vi "WPI_CAN_PDPGlobal.vi"(7 "Write After Receive":T2, 8 "Command":bool, 10 "Operation":T3, 11 "Power Distribution Panel (0)":u8) -> (0 "Commands":T1, 1 "Get All":T2, 3 "Power Distribution Panel Out":u8)   [LabVIEW 2017]
uses:
  <vilib>/Rock Robotics/WPI/CAN/PDP/WPI_CAN_PDPGlobalOps.ctl
  <vilib>/Rock Robotics/WPI/CAN/PDP/WPI_CAN_PDPGetAll.ctl
  <vilib>/Rock Robotics/WPI/CAN/PDP/WPI_CAN_PDPCommands.ctl
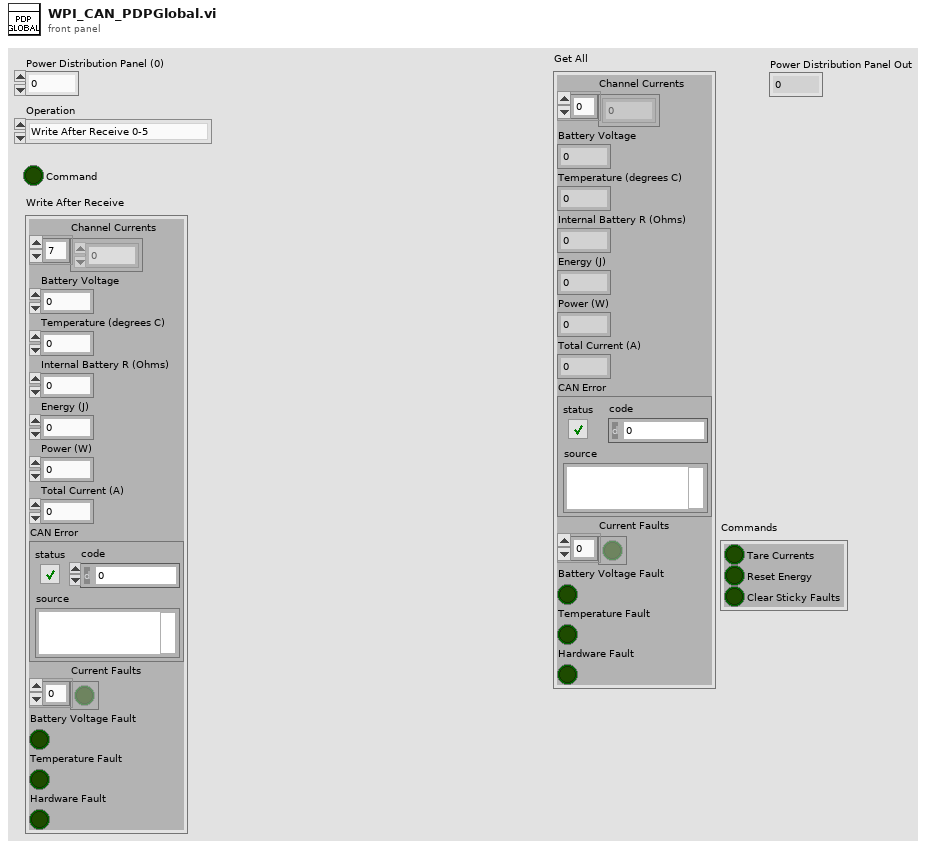
[diagram p1: front panel]
types:
  T1 = typedef "WPI_CAN_PDPCommands.ctl" = cluster{"Tare Currents":bool, "Reset Energy":bool, "Clear Sticky Faults":bool}
  T2 = typedef "WPI_CAN_PDPGetAll.ctl" = cluster{"Channel Currents":dbl[], "Battery Voltage":dbl, "Temperature (degrees C)":dbl, "Internal Battery R (Ohms)":dbl, "Energy (J)":dbl, "Power (W)":dbl, "Total Current (A)":dbl, "CAN Error":errorcluster, "Current Faults":bool[], "Battery Voltage Fault":bool, "Temperature Fault":bool, "Hardware Fault":bool}
  T3 = typedef "WPI_CAN_PDPGlobalOps.ctl" = enum16{"Write After Receive 0-5", "Write After Receive 6-11", "Write After Receive 12-15", "Write After Receive Energy", "Get All", "Get Commands", "Write Clear Sticky Faults Command", "Write Reset Energy Command", "Write Tare Currents Command", "Write Error", "Write After Receive Faults"}
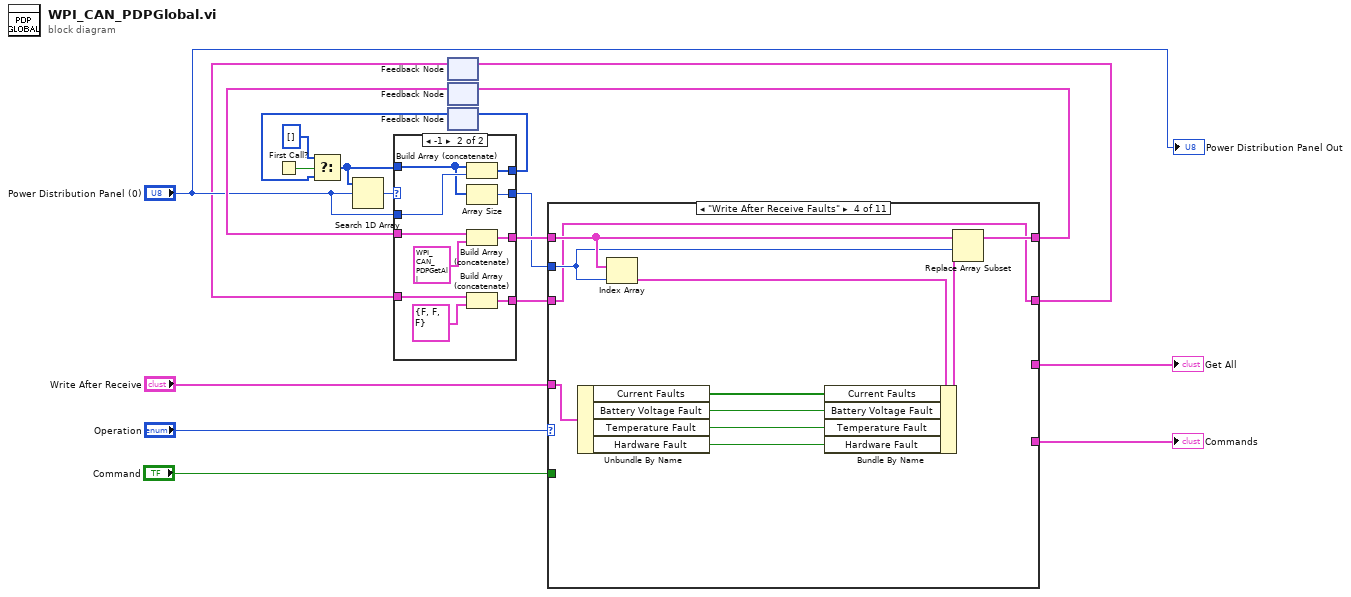
[diagram p0: block diagram]
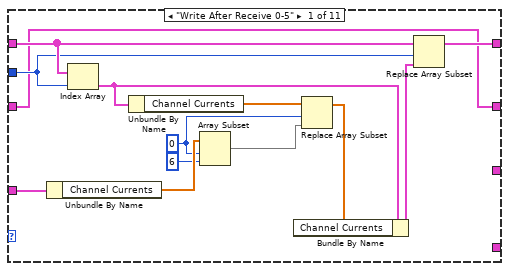
[diagram p2: hidden frame]
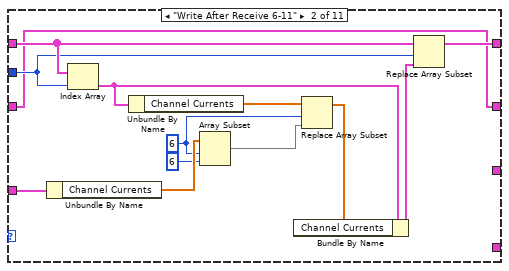
[diagram p3: hidden frame]
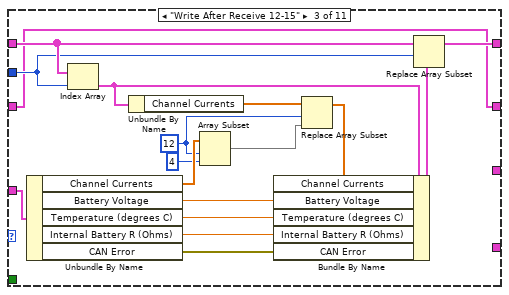
[diagram p4: hidden frame]
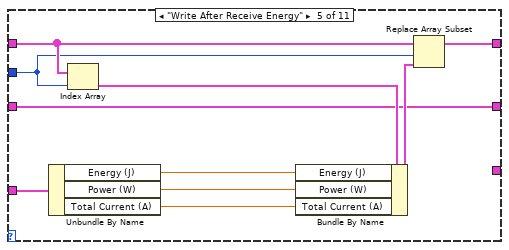
[diagram p5: hidden frame]
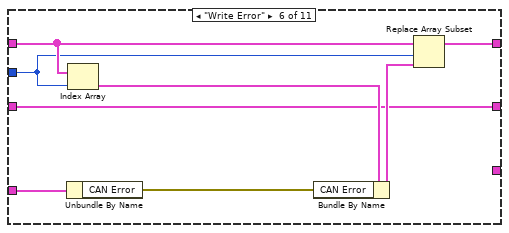
[diagram p6: hidden frame]
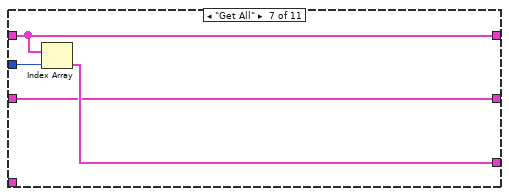
[diagram p7: hidden frame]
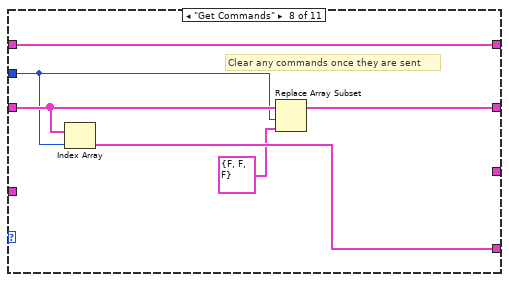
[diagram p8: hidden frame]
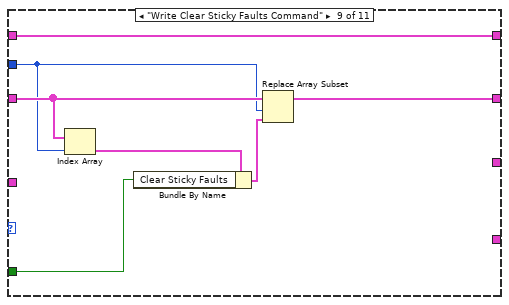
[diagram p9: hidden frame]
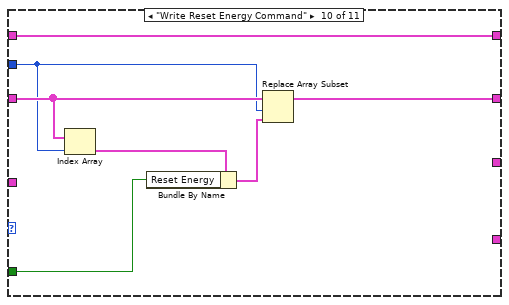
[diagram p10: hidden frame]
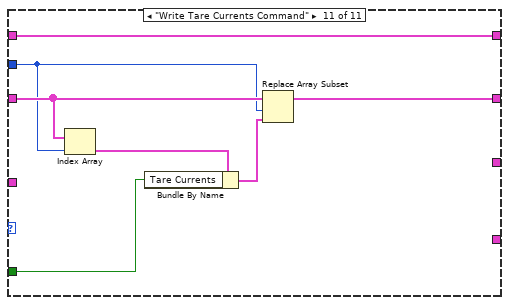
[diagram p11: hidden frame]
diagram:
  n1 = First Call?() -> (First Call?: T/F=w19:bool)
  n2 = feedback #1() -> (w3:T1[])  [unwired: 1 in]
  n3 = feedback #2() -> (w13:T2[])  [unwired: 1 in]
  n4 = feedback #3() -> (w17:u8[])  [unwired: 1 in]
  n5 = Select(t=u8[] [], s=w19, f=w17) -> (s? t:f=w15:u8[])
  n6 = Search 1D Array(1D array=w15, element="Power Distribution Panel (0)") -> (index of element=w14:i32)  [unwired: 1 in]
  n7 = case shown="-1" w14 {
    selector: w14 -> [w21 _]
    tunnel: [w23 w33] -> w16
    tunnel: "Power Distribution Panel (0)" -> [_ w32]
    tunnel: w15 -> [w23 w29]
    tunnel: w13 -> [w22 w31]
    tunnel: [w22 w30] -> w11
    tunnel: [w21 w28] -> w9
    tunnel: [w20 w25] -> w5
    tunnel: w3 -> [w20 w24]
    frame Default {
    }
    frame -1 {
      n8 = Build Array (concatenate)(w29, w32) -> (w33:u8[])
      n9 = Array Size(array=w29) -> (size(s)=w28:i32)
      n10 = Build Array (concatenate)(w31, T2 {"Channel Currents"=[0.0, 0.0, 0.0, 0.0, 0.0, 0.0, 0.0, 0.0, 0.0, 0.0, 0.0, 0.0, 0.0, 0.0, 0.0, 0.0], "Battery Voltage"=0.0, "Temperature (degrees C)"=0.0, "Internal Battery R (Ohms)"=0.0, "Energy (J)"=0.0, "Power (W)"=0.0, "Total Current (A)"=0.0, "CAN Error"={"status"=FALSE, "code"=0, "source"=""}, "Current Faults"=[], "Battery Voltage Fault"=FALSE, "Temperature Fault"=FALSE, "Hardware Fault"=FALSE} ("Write After Receive")) -> (w30:T2[])
      n11 = Build Array (concatenate)(w24, T1 {"Tare Currents"=FALSE, "Reset Energy"=FALSE, "Clear Sticky Faults"=FALSE} ("Commands")) -> (w25:T1[])
    }
  }
  n12 = feedback-in #3(w16) -> ()
  n13 = case shown="\"Write After Receive Faults\"" "Operation" {
    tunnel: [w46 w59 w76 w87 w97 w105 w108 w115 w122 w129 w136] -> w12
    tunnel: w11 -> [w45 w58 w75 w86 w96 w104 w108 w115 w122 w129 w136]
    tunnel: w9 -> [w44 w57 w74 w85 w95 w103 w109 w111 w119 w126 w133]
    tunnel: "Write After Receive" -> [w42 w55 w72 w83 w93 w101 _ _ _ _ _]
    tunnel: [_ _ _ _ _ _ w107 _ _ _ _] -> w7
    tunnel: [w34 w47 w60 w77 w88 w98 w106 w112 w121 w128 w135] -> w4
    tunnel: w5 -> [w34 w47 w60 w77 w88 w98 w106 w113 w120 w127 w134]
    tunnel: [_ _ _ _ _ _ _ w114 _ _ _] -> w2
    tunnel: "Command" -> [_ _ _ _ _ _ _ _ w116 w123 w130]
    frame "Write After Receive 0-5" {
      w36 = 0 ("length")
      n14 = Unbundle By Name(w42) -> ("Channel Currents"=w41:dbl[])
      n15 = Index Array(array=w45, index=w44) -> (element=w39:T2)
      n16 = Unbundle By Name(w39) -> ("Channel Currents"=w38:dbl[])
      n17 = Array Subset(array=w41, index=w36, length=6) -> (w35:dbl[])
      n18 = Replace Array Subset(array=w38, new element=w35, index=w36) -> (w37:dbl[])
      n19 = Bundle By Name(cluster=w39, "Channel Currents"=w37) -> (w43:T2)
      n20 = Replace Array Subset(array=w45, new element=w43, index=w44) -> (w46:T2[])
    }
    frame "Write After Receive 6-11" {
      w49 = 6 ("length")
      n21 = Unbundle By Name(w55) -> ("Channel Currents"=w54:dbl[])
      n22 = Index Array(array=w58, index=w57) -> (element=w52:T2)
      n23 = Unbundle By Name(w52) -> ("Channel Currents"=w51:dbl[])
      n24 = Array Subset(array=w54, index=w49, length=6) -> (w48:dbl[])
      n25 = Replace Array Subset(array=w51, new element=w48, index=w49) -> (w50:dbl[])
      n26 = Bundle By Name(cluster=w52, "Channel Currents"=w50) -> (w56:T2)
      n27 = Replace Array Subset(array=w58, new element=w56, index=w57) -> (w59:T2[])
    }
    frame "Write After Receive 12-15" {
      w65 = 12 ("length")
      n28 = Unbundle By Name(w72) -> ("Channel Currents"=w70:dbl[], "Battery Voltage"=w71:dbl, "Temperature (degrees C)"=w63:dbl, "Internal Battery R (Ohms)"=w62:dbl, "CAN Error"=w61:errorcluster)
      n29 = Index Array(array=w75, index=w74) -> (element=w68:T2)
      n30 = Unbundle By Name(w68) -> ("Channel Currents"=w67:dbl[])
      n31 = Array Subset(array=w70, index=w65, length=4) -> (w64:dbl[])
      n32 = Replace Array Subset(array=w67, new element=w64, index=w65) -> (w66:dbl[])
      n33 = Bundle By Name(cluster=w68, "Channel Currents"=w66, "Battery Voltage"=w71, "Temperature (degrees C)"=w63, "Internal Battery R (Ohms)"=w62, "CAN Error"=w61) -> (w73:T2)
      n34 = Replace Array Subset(array=w75, new element=w73, index=w74) -> (w76:T2[])
    }
    frame "Write After Receive Faults" {
      n35 = Unbundle By Name(w83) -> ("Current Faults"=w82:bool[], "Battery Voltage Fault"=w80:bool, "Temperature Fault"=w79:bool, "Hardware Fault"=w78:bool)
      n36 = Index Array(array=w86, index=w85) -> (element=w81:T2)
      n37 = Bundle By Name(cluster=w81, "Current Faults"=w82, "Battery Voltage Fault"=w80, "Temperature Fault"=w79, "Hardware Fault"=w78) -> (w84:T2)
      n38 = Replace Array Subset(array=w86, new element=w84, index=w85) -> (w87:T2[])
    }
    frame "Write After Receive Energy" {
      n39 = Unbundle By Name(w93) -> ("Energy (J)"=w91:dbl, "Power (W)"=w90:dbl, "Total Current (A)"=w89:dbl)
      n40 = Index Array(array=w96, index=w95) -> (element=w92:T2)
      n41 = Bundle By Name(cluster=w92, "Energy (J)"=w91, "Power (W)"=w90, "Total Current (A)"=w89) -> (w94:T2)
      n42 = Replace Array Subset(array=w96, new element=w94, index=w95) -> (w97:T2[])
    }
    frame "Write Error" {
      n43 = Unbundle By Name(w101) -> ("CAN Error"=w99:errorcluster)
      n44 = Index Array(array=w104, index=w103) -> (element=w100:T2)
      n45 = Bundle By Name(cluster=w100, "CAN Error"=w99) -> (w102:T2)
      n46 = Replace Array Subset(array=w104, new element=w102, index=w103) -> (w105:T2[])
    }
    frame "Get All" {
      n47 = Index Array(array=w108, index=w109) -> (element=w107:T2)
    }
    frame "Get Commands" {
      # "Clear any commands once they are sent"
      n48 = Index Array(array=w113, index=w111) -> (element=w114:T1)
      n49 = Replace Array Subset(array=w113, new element=T1 {"Tare Currents"=FALSE, "Reset Energy"=FALSE, "Clear Sticky Faults"=FALSE} ("Commands"), index=w111) -> (w112:T1[])
    }
    frame "Write Clear Sticky Faults Command" {
      n50 = Index Array(array=w120, index=w119) -> (element=w118:T1)
      n51 = Bundle By Name(cluster=w118, "Clear Sticky Faults"=w116) -> (w117:T1)
      n52 = Replace Array Subset(array=w120, new element=w117, index=w119) -> (w121:T1[])
    }
    frame "Write Reset Energy Command" {
      n53 = Index Array(array=w127, index=w126) -> (element=w125:T1)
      n54 = Bundle By Name(cluster=w125, "Reset Energy"=w123) -> (w124:T1)
      n55 = Replace Array Subset(array=w127, new element=w124, index=w126) -> (w128:T1[])
    }
    frame "Write Tare Currents Command" {
      n56 = Index Array(array=w134, index=w133) -> (element=w132:T1)
      n57 = Bundle By Name(cluster=w132, "Tare Currents"=w130) -> (w131:T1)
      n58 = Replace Array Subset(array=w134, new element=w131, index=w133) -> (w135:T1[])
    }
  }
  "Get All" <- w7
  "Commands" <- w2
  n59 = feedback-in #1(w4) -> ()
  n60 = feedback-in #2(w12) -> ()
  "Power Distribution Panel Out" <- "Power Distribution Panel (0)"
